vi "sub_lookahead_calculate.vi"() -> (0 "center point":cluster{"x":dbl, "y":dbl} {"x" format="%.2f"; "y" format="%.2f"}, 1 "looktail":cluster{"x":dbl, "y":dbl} {"x" format="%.2f"; "y" format="%.2f"}, 2 "lookahead":cluster{"x":dbl, "y":dbl} {"x" format="%.2f"; "y" format="%.2f"}, 3 "agv lookahead circle":cluster{"x":dbl, "y":dbl}[](array[cluster]) {"x" format="%.2f"; "y" format="%.2f"}, 5 "deg_wpts gps-base":dbl)   [LabVIEW 2019]
uses:
  Ctrl/waypoint_buf.ctl
  Ctrl/pid-in-params.ctl
  Ctrl/points.ctl
  <vilib>/gmath/NI_Gmath.lvlib
panel:
  out "true tail":cluster{"x":dbl, "y":dbl}
  out "크기":i32
  out "XY 그래프":cluster{cluster{dbl, dbl}[]}[](graph)
  out "slope":dbl
  out "virtual waypoints":cluster{"x":dbl, "y":dbl}[](array[cluster]) {"x" format="%.2f"; "y" format="%.2f"}
  out "dis graph":dbl[](graph)
  out "in circle waypts":cluster{"x":dbl, "y":dbl}[](array[cluster]) {"x" format="%.2f"; "y" format="%.2f"}
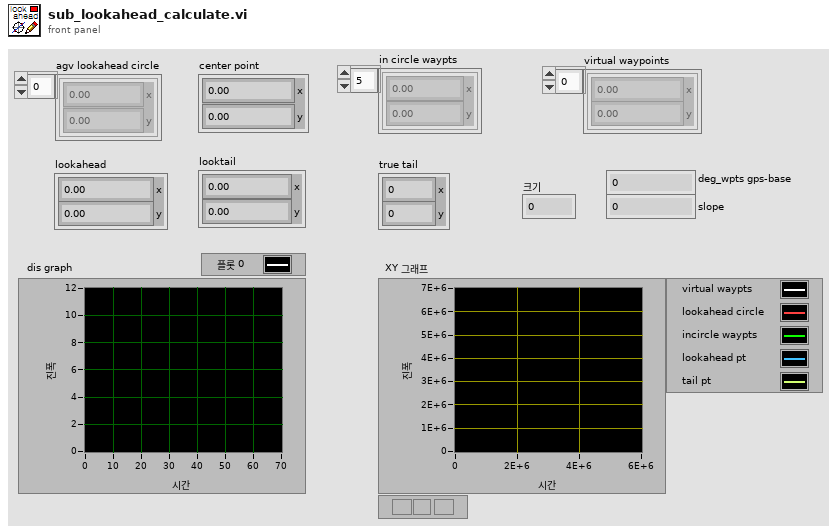
[diagram p1: front panel]
types:
  T1 = typedef "waypoint_buf.ctl" = enum16{"clear", "write", "read"}
  T2 = cluster{"lookahead pt n":dbl, "lookahead distance":dbl}
  T3 = typedef "pid-in-params.ctl" = enum16{"read", "write"}
  T4 = cluster{"deg_agv-lookahead":dbl, "deg_waypoint":dbl, "deg_gap":dbl, "deg_target":dbl, "pid output":dbl, "distance-gap_out":dbl}
  T5 = typedef "points.ctl" = enum16{"read", "lookahead circle in", "lookahead in", "looktail in", "center in"}
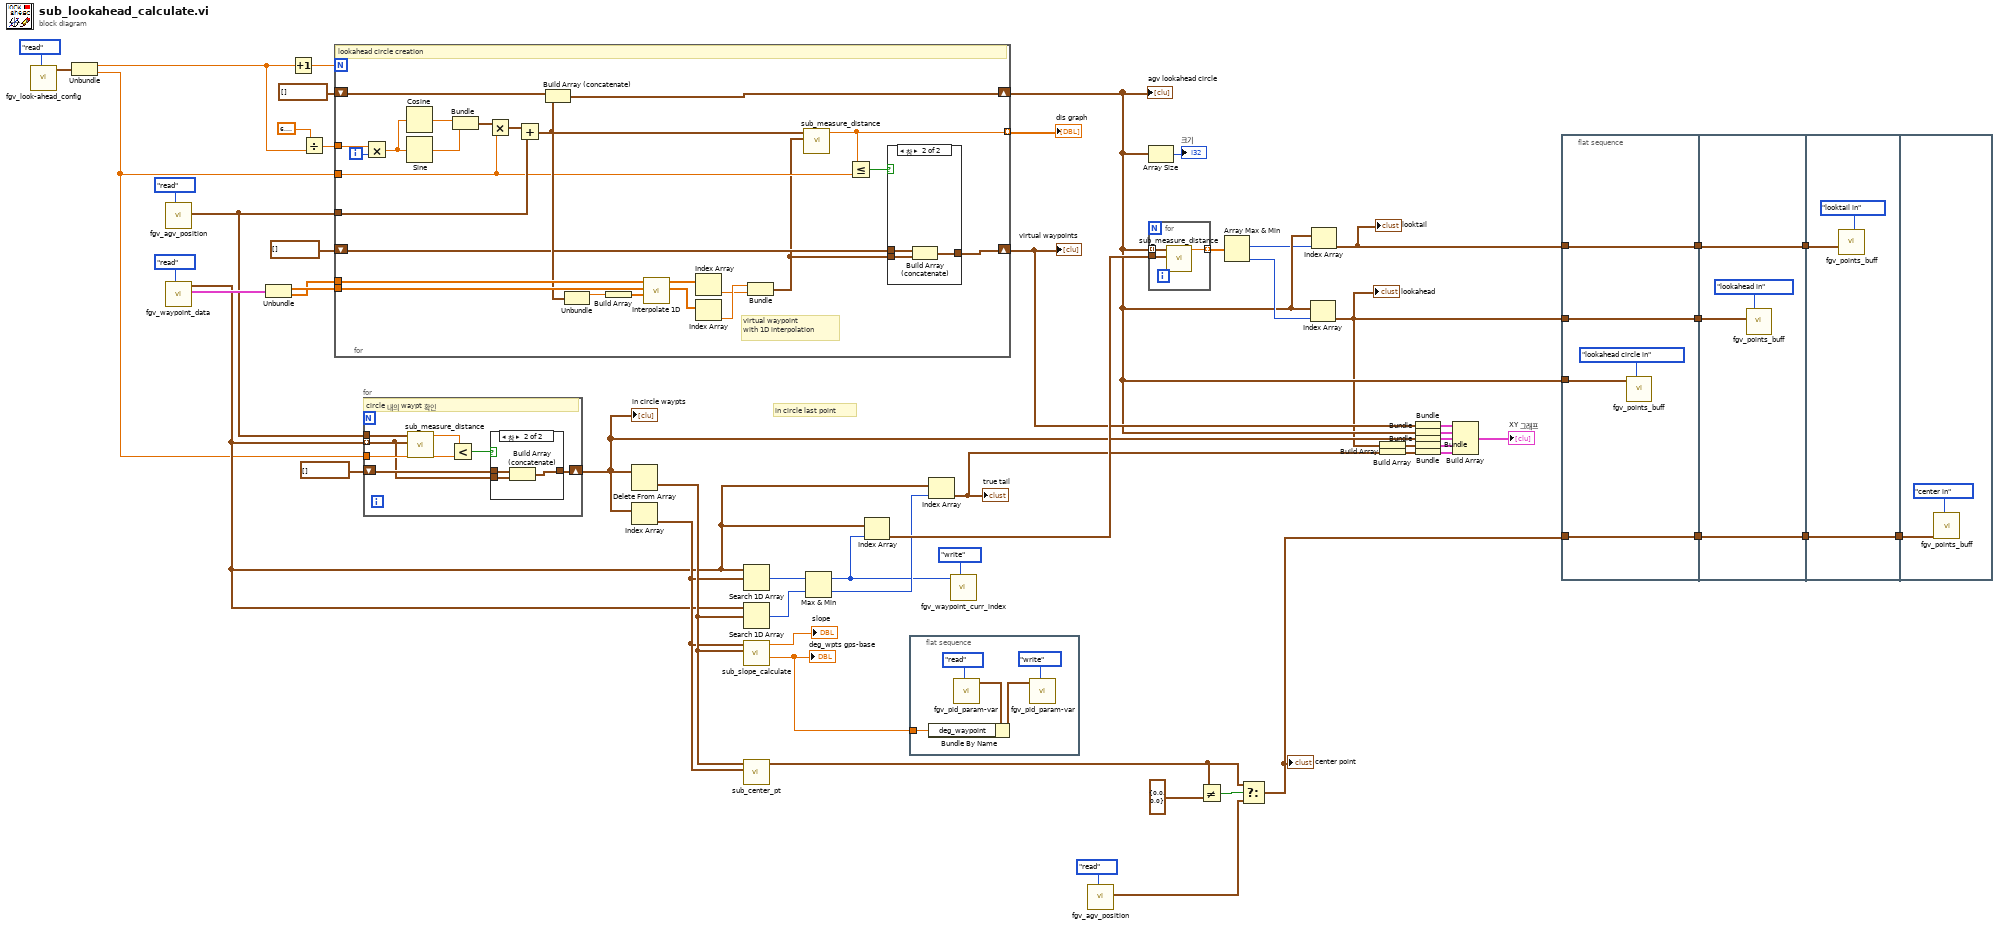
[diagram p0: block diagram]
diagram:
  # "in circle last point"
  n1 = call "fgv_look-ahead_config.vi"("cmd"=enum16{"read", "write"}."read") -> ("lookahed cfg out"=w31:T2)  [unwired: 10 in]
  n2 = Unbundle(w31) -> ("lookahead pt n"=w32:dbl, "lookahead distance"=w12:dbl)
  n3 = call "fgv_agv_position.vi"("cmd"=enum16{"write", "read"}."read") -> ("utm out"=w1:cluster{dbl, dbl})  [unwired: 8 in, 2 out]
  n4 = call "fgv_waypoint_data.vi"("cmd"=waypoint_buf."read") -> ("xy-arrys out"=w55:cluster{"x array":dbl[], "y arrays":dbl[]}, "waypoint out"=w23:cluster{"x":dbl, "y":dbl}[])  [unwired: 8 in, 1 out]
  n5 = Unbundle(w55) -> ("x array"=w57:dbl[], "y arrays"=w56:dbl[])
  n6 = Increment(x=w32) -> (x+1=w54:dbl)
  n7 = Divide(x=6.283185307179586, y=w32) -> (x/y=w51:dbl)
  n8 = for {
    N: w54 -> [_]
    shift-right: [w80] -> w21
    shift-left: cluster{dbl, dbl}[] [] -> [w79]
    tunnel: w51 -> [w82]
    tunnel: w1 -> [w66]
    tunnel: w56 -> [w76]
    tunnel: w57 -> [w75]
    tunnel: [w59] -> w50 mode=indexing
    tunnel: w12 -> [w64]
    shift-right: [w62] -> w40
    shift-left: cluster{dbl, dbl}[] [] -> [w61]
    i -> [w83]
    # "virtual waypoint\nwith 1D interpolation"
    # "lookahead circle creation"
    n9 = Multiply(x=w82, y=w83) -> (x*y=w81:dbl)
    n10 = Cosine(x=w81) -> (cos(x)=w70:dbl)
    n11 = Sine(x=w81) -> (sin(x)=w69:dbl)
    n12 = Bundle(w70, w69) -> (w78:cluster{dbl, dbl})  [unwired: 1 in]
    n13 = Multiply(x=w78, y=w64) -> (x*y=w77:cluster{dbl, dbl})
    n14 = Add(x=w77, y=w66) -> (x+y=w65:cluster{dbl, dbl})
    n15 = Build Array (concatenate)(w79, w65) -> (w80:cluster{dbl, dbl}[])
    n16 = Unbundle(w65) -> (w71:dbl)  [unwired: 1 out]
    n17 = Build Array(w71) -> (w74:dbl[])
    n18 = call <vilib>:"Interpolate 1D.vi"("xi"=w74, "X"=w75, "Y"=w76) -> ("xi used"=w72:dbl[], "yi"=w73:dbl[])  [unwired: 6 in, 1 out]
    n19 = Index Array(array=w73) -> (element=w67:dbl)  [unwired: 1 in]
    n20 = Index Array(array=w72) -> (element=w68:dbl)  [unwired: 1 in]
    n21 = Bundle("Numeric"=w68, "Numeric"=w67) -> (w60:cluster{"Numeric":dbl, "Numeric":dbl})  [unwired: 1 in]
    n22 = call "sub_measure_distance.vi"("pt 2"=w60, "pt 1"=w65) -> ("distance"=w59:dbl)  [unwired: 9 in]
    n23 = Less Or Equal?(x=w59, y=w64) -> (x <= y?=w63:bool)
    n24 = case shown="참" w63 {
      tunnel: [w84 w87] -> w62
      tunnel: w61 -> [w84 w86]
      tunnel: w60 -> [_ w85]
      frame False {
      }
      frame True {
        n25 = Build Array (concatenate)(w86, w85) -> (w87:cluster{"Numeric":dbl, "Numeric":dbl}[])
      }
    }
  }
  "agv lookahead circle" <- w21
  "dis graph" <- w50
  "virtual waypoints" <- w40
  n26 = for {
    tunnel: w23 -> [w89] mode=indexing
    tunnel: w1 -> [w94]
    shift-right: [w88] -> w35
    shift-left: cluster{"x":dbl, "y":dbl}[] [] -> [w91]
    tunnel: w12 -> [w92]
    # "circle 내의 waypt 확인"
    n27 = call "sub_measure_distance.vi"("pt 2"=w89, "pt 1"=w94) -> ("distance"=w93:dbl)  [unwired: 9 in]
    n28 = Less?(x=w93, y=w92) -> (x < y?=w90:bool)
    n29 = case shown="참" w90 {
      tunnel: w91 -> [w95 w98]
      tunnel: w89 -> [_ w97]
      tunnel: [w95 w96] -> w88
      frame False {
      }
      frame True {
        n30 = Build Array (concatenate)(w98, w97) -> (w96:cluster{"x":dbl, "y":dbl}[])
      }
    }
  }
  "in circle waypts" <- w35
  n31 = Delete From Array(array=w35) -> (deleted portion=w34:cluster{"x":dbl, "y":dbl})  [unwired: 2 in, 1 out]
  n32 = Index Array(array=w35) -> (element=w33:cluster{"x":dbl, "y":dbl})  [unwired: 1 in]
  n33 = Search 1D Array(1D array=w23, element=w33) -> (index of element=w47:i32)  [unwired: 1 in]
  n34 = Search 1D Array(1D array=w23, element=w34) -> (index of element=w46:i32)  [unwired: 1 in]
  n35 = call "sub_slope_calculate.vi"("point n+1"=w34, "point n"=w33) -> ("deg_gps-base"=w11:dbl, "slope"=→"slope":dbl)  [unwired: 7 in, 1 out]
  "deg_wpts gps-base" <- w11
  n36 = call "sub_center_pt.vi"("point-2"=w33, "point-1"=w34) -> ("center"=w5:cluster{"x":dbl, "y":dbl})  [unwired: 9 in]
  n37 = Max & Min(x=w47, y=w46) -> (max(x,y)=w10:i32, min(x,y)=w22:i32)
  n38 = Index Array(array=w23, index=w10) -> (element=w41:cluster{"x":dbl, "y":dbl})
  n39 = flat-sequence {
    tunnel: w11 -> [w99]
    frame #0 {
      n40 = call "fgv_pid_param-var.vi"("cmd"=pid-in-params."read") -> ("pid-var_output"=w101:T4)  [unwired: 10 in]
      n41 = Bundle By Name(cluster=w101, "deg_waypoint"=w99) -> (w100:T4)
      n42 = call "fgv_pid_param-var.vi"("cmd"=pid-in-params."write", "pid-vars_in"=w100) -> ()  [unwired: 9 in, 1 out]
    }
  }
  n43 = Index Array(array=w23, index=w22) -> (element=w18:cluster{"x":dbl, "y":dbl})
  "true tail" <- w18
  n44 = call "fgv_waypoint_curr_index.vi"("cmd"=enum16{"write", "read"}."write", "index in"=w10) -> ()  [unwired: 9 in, 1 out]
  n45 = call "fgv_agv_position.vi"("cmd"=enum16{"write", "read"}."read") -> ("utm out"=w2:cluster{dbl, dbl})  [unwired: 8 in, 2 out]
  n46 = Array Size(array=w21) -> (size(s)=→"크기":i32)
  n47 = for {
    tunnel: w21 -> [w106] mode=indexing
    tunnel: w41 -> [w105]
    tunnel: [w104] -> w45 mode=indexing
    n48 = call "sub_measure_distance.vi"("pt 2"=w105, "pt 1"=w106) -> ("distance"=w104:dbl)  [unwired: 9 in]
  }
  n49 = Not Equal?(x=w5, y=cluster{"x":dbl, "y":dbl} {"x"=0.0, "y"=0.0} ("center")) -> (x != y?=w6:bool)
  n50 = Array Max & Min(array=w45) -> (max index (indices)=w20:i32, min index (indices)=w44:i32)  [unwired: 2 out]
  n51 = Select(t=w5, s=w6, f=w2) -> (s? t:f=w3:cluster{"x":dbl, "y":dbl})
  "center point" <- w3
  n52 = Index Array(array=w21, index=w44) -> (element=w16:cluster{dbl, dbl})
  "lookahead" <- w16
  n53 = Index Array(array=w21, index=w20) -> (element=w19:cluster{dbl, dbl})
  "looktail" <- w19
  n54 = Build Array(w16) -> (w15:cluster{dbl, dbl}[])
  n55 = Build Array(w18) -> (w17:cluster{"x":dbl, "y":dbl}[])
  n56 = Bundle(w40) -> (w39:cluster{cluster{dbl, dbl}[]})  [unwired: 1 in]
  n57 = Bundle(w21) -> (w37:cluster{cluster{dbl, dbl}[]})  [unwired: 1 in]
  n58 = Bundle(w35) -> (w36:cluster{cluster{"x":dbl, "y":dbl}[]})  [unwired: 1 in]
  n59 = Bundle(w15) -> (w14:cluster{cluster{dbl, dbl}[]})  [unwired: 1 in]
  n60 = Bundle(w17) -> (w13:cluster{cluster{"x":dbl, "y":dbl}[]})  [unwired: 1 in]
  n61 = Build Array(w39, w37, w36, w14, w13) -> (→"XY 그래프":cluster{cluster{"x":dbl, "y":dbl}[]}[])
  n62 = flat-sequence {
    tunnel: w21 -> [w110]
    tunnel: [w109] -> w30
    tunnel: w16 -> [w109]
    tunnel: w19 -> [w108]
    tunnel: [w108] -> w29
    tunnel: w3 -> [w107]
    tunnel: [w107] -> w27
    tunnel: w30 -> [w114]
    tunnel: w29 -> [w113]
    tunnel: [w113] -> w28
    tunnel: w27 -> [w112]
    tunnel: [w112] -> w26
    tunnel: w28 -> [w117]
    tunnel: w26 -> [w116]
    tunnel: [w116] -> w25
    tunnel: w25 -> [w119]
    frame #0 {
      n63 = call "fgv_points_buff.vi"("cmd"=points."lookahead circle in", "lookahead circle in"=w110) -> ()  [unwired: 6 in, 4 out]
    }
    frame #1 {
      n64 = call "fgv_points_buff.vi"("cmd"=points."lookahead in", "lookahead in"=w114) -> ()  [unwired: 6 in, 4 out]
    }
    frame #2 {
      n65 = call "fgv_points_buff.vi"("cmd"=points."looktail in", "looktail in"=w117) -> ()  [unwired: 6 in, 4 out]
    }
    frame #3 {
      n66 = call "fgv_points_buff.vi"("cmd"=points."center in", "center in"=w119) -> ()  [unwired: 6 in, 4 out]
    }
  }
